vi "DIM_DIO.destructor.vi"(0 "i ref in":refnum<vi>, 5 "error in (no error)":errorcluster) -> (19 "error out":errorcluster)   [LabVIEW 2014, in "DIM_DIO.lvlib"]
doc: "This is the destructor of a class.\n\nLicense Agreement for this software:\n\nCopyright (C)\nGesellschaft für Schwerionenforschung, GSI\nPlanckstr. 1\n64291 Darmstadt\nGermany\n\nContact: D.Beck@gsi.de \n\nThis program is free software; you can redistribute it and/or modify it under the terms of the \nGNU General Public License as published by the Free Software Foundation; either version 2 of \nthe license, or (at your option) any later version.\n\nThis program is distributed in the hope that it will be useful, but WITHOUT ANY WARRANTY; \nwithout even the implied warranty of MERCHANTABILITY or FITNESS FOR A PARTICULAR PURPOSE. See the GNU General License for more details (http://www.gnu.org).\n\nGesellschaft für Schwerionenforschung, GSI\nPlanckstr. 1, 64291 Darmstadt, Germany\nFor all questions and ideas contact: M.Richter@gsi.de, H.Brand@gsi.de or D.Beck@gsi.de.\nLast update: 16-JUN-2004"
uses:
  DIM_DIO.lvlib
  CSlibraries-extern/DimLVEvent/LVDimInterface/LVDimInterface.lvlib
  CS_Core/CSApplicationBaseClasses/DigiIOBase/DigiIOBase.lvlib
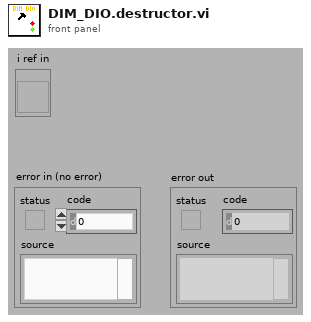
[diagram p1: front panel]
types:
  T1 = typedef "DIM_DIO.lvlib/DIM_DIO.i attribute.ctl" = cluster{"serviceIDs":cluster{"writeBitID":i32}}
  T2 = enum16{"SetAttribute", "GetAttribute", "CreateAttribute", "DestroyAttribute", "DestroyAllAtributes"}
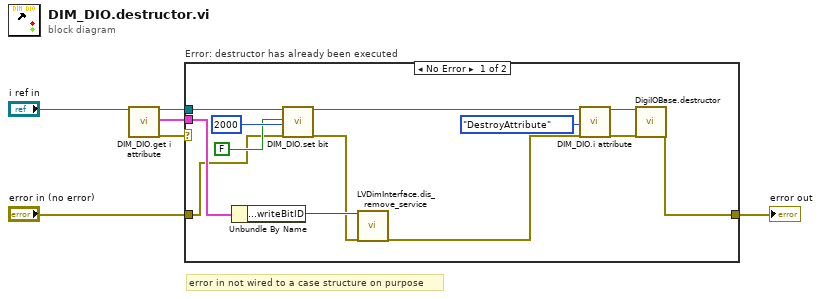
[diagram p0: block diagram]
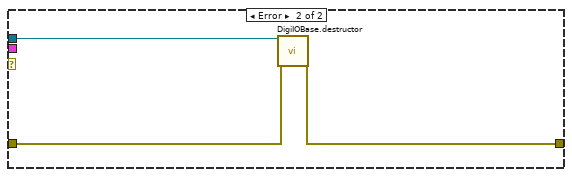
[diagram p2: hidden frame]
diagram:
  # "error in not wired to a case structure on purpose"
  n1 = call "DIM_DIO.get i attribute.vi"("i ref in"="i ref in") -> ("i ref out"=w3:refnum<vi>, "i attribute"=w1:T1, "error out"=w2:errorcluster)  [unwired: 16 in]
  n2 = case "Error: destructor has already been executed" shown="No Error" w2 {
    tunnel: [w16 w20] -> w6
    tunnel: "error in (no error)" -> [w7 w21]
    tunnel: w3 -> [w15 w22]
    tunnel: w1 -> [w12 _]
    frame No Error {
      n3 = Unbundle By Name(w12) -> ("serviceIDs.writeBitID"=w11:i32)
      n4 = call "DIM_DIO.set bit.vi"("i ref in"=w15, "bitValue"=FALSE, "ms timeout (10000)"=2000, "error in (no error)"=w7) -> ("i ref out"=w9:refnum<vi>, "error out"=w10:errorcluster)  [unwired: 13 in, 1 out]
      n5 = call "LVDimInterface.dis_remove_service.vi"("my_serviceID"=w11, "error in (no error)"=w10) -> ("error out"=w8:errorcluster)  [unwired: 17 in]
      n6 = call "DIM_DIO.i attribute.vi"("VI Refnum"=w9, "Action"=T2."DestroyAttribute", "error in (no error)"=w8) -> ("VI Refnum out"=w18:refnum<vi>, "error out"=w17:errorcluster)  [unwired: 14 in, 1 out]
      n7 = call "DigiIOBase.destructor.vi"("i ref in"=w18, "error in (no error)"=w17) -> ("error out"=w16:errorcluster)  [unwired: 17 in]
    }
    frame Error {
      n8 = call "DigiIOBase.destructor.vi"("i ref in"=w22, "error in (no error)"=w21) -> ("error out"=w20:errorcluster)  [unwired: 17 in]
    }
  }
  "error out" <- w6
